vi "Lab Panel V5.23.vi"() -> ()   [LabVIEW 2013] (continued)
                    n2880 = Number To Decimal String(number=w5323) -> (decimal integer string=w5325:string)  [unwired: 1 in]
                    n2881 = Number To Decimal String(number=w5320) -> (decimal integer string=w5318:string)  [unwired: 1 in]
                    n2882 = Number To Decimal String(number=w5315) -> (decimal integer string=w5313:string)  [unwired: 1 in]
                    n2883 = Number To Decimal String(number=w5330) -> (decimal integer string=w5328:string)  [unwired: 1 in]
                    n2884 = Number To Decimal String(number=w5310) -> (decimal integer string=w5308:string)  [unwired: 1 in]
                    n2885 = Number To Decimal String(number=w5335) -> (decimal integer string=w5333:string)  [unwired: 1 in]
                    n2886 = Number To Decimal String(number=w5337) -> (decimal integer string=w5290:string)  [unwired: 1 in]
                    n2887 = Number To Decimal String(number=w5305) -> (decimal integer string=w5303:string)  [unwired: 1 in]
                    n2888 = Number To Decimal String(number=w5300) -> (decimal integer string=w5298:string)  [unwired: 1 in]
                    n2889 = Number To Decimal String(number=w5295) -> (decimal integer string=w5293:string)  [unwired: 1 in]
                    n2890 = Number To Fractional String(number=w5322, precision (6)=w5267) -> (F-format string=w5324:string)  [unwired: 2 in]
                    n2891 = Number To Fractional String(number=w5309, precision (6)=w5267) -> (F-format string=w5307:string)  [unwired: 2 in]
                    n2892 = Number To Fractional String(number=w5319, precision (6)=w5267) -> (F-format string=w5317:string)  [unwired: 2 in]
                    n2893 = Number To Fractional String(number=w5314, precision (6)=w5267) -> (F-format string=w5312:string)  [unwired: 2 in]
                    n2894 = Number To Fractional String(number=w5299, precision (6)=w5267) -> (F-format string=w5297:string)  [unwired: 2 in]
                    n2895 = Number To Fractional String(number=w5304, precision (6)=w5267) -> (F-format string=w5302:string)  [unwired: 2 in]
                    n2896 = Number To Fractional String(number=w5329, precision (6)=w5267) -> (F-format string=w5327:string)  [unwired: 2 in]
                    n2897 = Number To Fractional String(number=w5294, precision (6)=w5267) -> (F-format string=w5292:string)  [unwired: 2 in]
                    n2898 = Number To Fractional String(number=w5334, precision (6)=w5267) -> (F-format string=w5332:string)  [unwired: 2 in]
                    n2899 = Number To Fractional String(number=w5336, precision (6)=w5267) -> (F-format string=w5289:string)  [unwired: 2 in]
                    n2900 = Concatenate Strings(w5266, w5308, w5266, w5307, w5266, w5306) -> (w5282:string)
                    n2901 = Concatenate Strings(w5266, w5303, w5266, w5302, w5266, w5301) -> (w5281:string)
                    n2902 = Concatenate Strings(w5266, w5298, w5266, w5297, w5266, w5296) -> (w5280:string)
                    n2903 = Concatenate Strings(w5266, w5293, w5266, w5292, w5266, w5291) -> (w5279:string)
                    n2904 = Concatenate Strings(w5266, w5290, w5266, w5289, w5266, w5288) -> (w5278:string)
                    n2905 = Concatenate Strings(w5266, w5333, w5266, w5332, w5266, w5331) -> (w5287:string)
                    n2906 = Concatenate Strings(w5266, w5313, w5266, w5312, w5266, w5311) -> (w5283:string)
                    n2907 = Concatenate Strings(w5266, w5328, w5266, w5327, w5266, w5326) -> (w5286:string)
                    n2908 = Concatenate Strings(w5266, w5325, w5266, w5324, w5266, w5321) -> (w5285:string)
                    n2909 = Concatenate Strings(w5266, w5318, w5266, w5317, w5266, w5316) -> (w5284:string)
                    n2910 = Concatenate Strings("]", "\r") -> (w5263:string)
                    n2911 = Concatenate Strings(w5258, w5283, w5263) -> (w5273:string)
                    n2912 = Concatenate Strings(w5260, w5285, w5263) -> (w5275:string)
                    n2913 = Concatenate Strings(w5259, w5284, w5263) -> (w5274:string)
                    n2914 = Concatenate Strings(w5255, w5280, w5263) -> (w5270:string)
                    n2915 = Concatenate Strings(w5256, w5279, w5263) -> (w5271:string)
                    n2916 = Concatenate Strings(w5254, w5281, w5263) -> (w5269:string)
                    n2917 = Concatenate Strings(w5253, w5282, w5263) -> (w5268:string)
                    n2918 = Concatenate Strings(w5257, w5278, w5263) -> (w5272:string)
                    n2919 = Concatenate Strings(w5261, w5286, w5263) -> (w5276:string)
                    n2920 = Concatenate Strings(w5262, w5287, w5263) -> (w5277:string)
                    n2921 = Concatenate Strings(w5277, w5276, w5275, w5274, w5273, w5268, w5269, w5270, w5271, w5272) -> (w5246:string)
                    n2922 = Concatenate Strings("[PANEL/", "DESC/", "CYCLES/", "MINS/", "STATUS]", "\r", w5246) -> (w5245:string)
                    "MAIL REPORT" <- w5245
                    n2923 = global write "Global display 3.vi" "log all"(w5245) -> ()
                  }
                  frame #2 {
                    w5376 = "END"
                    n2924 = local read "mail control"() -> (w5377:string)
                    n2925 = case shown="False" w5372 {
                      tunnel: w5377 -> [w5401 _]
                      tunnel: w5376 -> [w5400 _]
                      tunnel: [w5399 FALSE] -> w5362
                      frame False {
                        n2926 = Equal?(x=w5401, y=w5400) -> (x = y?=w5399:bool)
                      }
                      frame True {
                      }
                    }
                    n2927 = case shown="False" w5378 {
                      tunnel: w5377 -> [w5417 _]
                      tunnel: w5376 -> [w5416 _]
                      tunnel: [w5415 FALSE] -> w5366
                      frame False {
                        n2928 = Equal?(x=w5417, y=w5416) -> (x = y?=w5415:bool)
                      }
                      frame True {
                      }
                    }
                    n2929 = case shown="False" w5375 {
                      tunnel: w5377 -> [w5413 _]
                      tunnel: w5376 -> [w5412 _]
                      tunnel: [w5411 FALSE] -> w5365
                      frame False {
                        n2930 = Equal?(x=w5413, y=w5412) -> (x = y?=w5411:bool)
                      }
                      frame True {
                      }
                    }
                    n2931 = case shown="False" w5373 {
                      tunnel: w5377 -> [w5405 _]
                      tunnel: w5376 -> [w5404 _]
                      tunnel: [w5403 FALSE] -> w5363
                      frame False {
                        n2932 = Equal?(x=w5405, y=w5404) -> (x = y?=w5403:bool)
                      }
                      frame True {
                      }
                    }
                    n2933 = case shown="False" w5374 {
                      tunnel: w5377 -> [w5409 _]
                      tunnel: w5376 -> [w5408 _]
                      tunnel: [w5407 FALSE] -> w5364
                      frame False {
                        n2934 = Equal?(x=w5409, y=w5408) -> (x = y?=w5407:bool)
                      }
                      frame True {
                      }
                    }
                    n2935 = Or(x=w5364, y=w5363) -> (x .or. y?=w5355:bool)
                    n2936 = Or(x=w5366, y=w5365) -> (x .or. y?=w5356:bool)
                    n2937 = Or(x=w5356, y=w5355) -> (x .or. y?=w5351:bool)
                    n2938 = case shown="False" w5368 {
                      tunnel: w5377 -> [w5385 _]
                      tunnel: w5376 -> [w5384 _]
                      tunnel: [w5383 FALSE] -> w5357
                      frame False {
                        n2939 = Equal?(x=w5385, y=w5384) -> (x = y?=w5383:bool)
                      }
                      frame True {
                      }
                    }
                    n2940 = case shown="False" w5367 {
                      tunnel: w5377 -> [w5381 _]
                      tunnel: w5376 -> [w5380 _]
                      tunnel: [w5379 FALSE] -> w5361
                      frame False {
                        n2941 = Equal?(x=w5381, y=w5380) -> (x = y?=w5379:bool)
                      }
                      frame True {
                      }
                    }
                    n2942 = case shown="False" w5369 {
                      tunnel: w5377 -> [w5389 _]
                      tunnel: w5376 -> [w5388 _]
                      tunnel: [w5387 FALSE] -> w5358
                      frame False {
                        n2943 = Equal?(x=w5389, y=w5388) -> (x = y?=w5387:bool)
                      }
                      frame True {
                      }
                    }
                    n2944 = case shown="False" w5371 {
                      tunnel: w5377 -> [w5397 _]
                      tunnel: w5376 -> [w5396 _]
                      tunnel: [w5395 FALSE] -> w5360
                      frame False {
                        n2945 = Equal?(x=w5397, y=w5396) -> (x = y?=w5395:bool)
                      }
                      frame True {
                      }
                    }
                    n2946 = case shown="False" w5370 {
                      tunnel: w5377 -> [w5393 _]
                      tunnel: w5376 -> [w5392 _]
                      tunnel: [w5391 FALSE] -> w5359
                      frame False {
                        n2947 = Equal?(x=w5393, y=w5392) -> (x = y?=w5391:bool)
                      }
                      frame True {
                      }
                    }
                    n2948 = Or(x=w5360, y=w5359) -> (x .or. y?=w5354:bool)
                    n2949 = Or(x=w5358, y=w5357) -> (x .or. y?=w5353:bool)
                    n2950 = Or(x=w5361, y=w5362) -> (x .or. y?=w5349:bool)
                    n2951 = Or(x=w5354, y=w5353) -> (x .or. y?=w5352:bool)
                    n2952 = Or(x=w5351, y=w5352) -> (x .or. y?=w5350:bool)
                    n2953 = Or(x=w5350, y=w5349) -> (x .or. y?=w5348:bool)
                  }
                  frame #3 {
                    n2954 = local read "on loops"() -> (w5431:dbl)
                    n2955 = local read "jig cycle"() -> (w5428:dbl)
                    n2956 = local read "Send Mail Now"() -> (w5422:bool)
                    n2957 = Add(x=w5431, y=3.0) -> (x+y=w5429:dbl)
                    n2958 = Equal?(x=w5428, y=w5429) -> (x = y?=w5423:bool)
                    n2959 = And(x=w5423, y=w5422) -> (x .and. y?=w5421:bool)
                    n2960 = And(x=w5427, y=w5423) -> (x .and. y?=w5426:bool)
                    n2961 = And(x=w5426, y=w5425) -> (x .and. y?=w5424:bool)
                    n2962 = Or(x=w5424, y=w5421) -> (x .or. y?=w5420:bool)
                    n2963 = case shown="True" w5420 {
                      tunnel: w5436 -> [_ w5442]
                      tunnel: w5435 -> [_ w5441]
                      tunnel: "Lab Panel Test Status" -> [_ w5440]
                      tunnel: w5433 -> [_ w5439]
                      tunnel: w5432 -> [_ w5438]
                      tunnel: w5419 -> [_ w5437]
                      frame False {
                      }
                      frame True {
                        n2964 = stacked-sequence {
                          tunnel: w5442 -> [w5450 _]
                          tunnel: w5441 -> [w5449 _]
                          tunnel: w5440 -> [w5448 _]
                          tunnel: w5439 -> [w5447 _]
                          tunnel: w5438 -> [w5446 _]
                          tunnel: w5437 -> [w5445 _]
                          frame #0 {
                            n2965 = call "sub vi - send mail v5.vi"("TO:"=w5450, "subject"=w5448, "from"=w5446, "out going server"=w5447, "message"=w5449) -> ("error out"=w5444:errorcluster)  [unwired: 10 in]
                            n2966 = Bundle(cluster=w5445, "mail error"=w5444) -> (w5443:T7)  [unwired: 6 in]
                            n2967 = local write "MAIL SETTINGS"(w5443) -> ()
                          }
                          frame #1 {
                            n2968 = local write "mail control"("") -> ()
                            n2969 = local write "Send Mail Now"(FALSE) -> ()
                          }
                        }
                      }
                    }
                  }
                }
              }
            }
          }
          frame #18 {
            # "save jig cycle values once all run switches are off"
            n2970 = stacked-sequence {
              tunnel: w5462 -> [_ w5491]
              tunnel: w5461 -> [_ w5490]
              tunnel: w5460 -> [_ w5489]
              tunnel: w5459 -> [_ w5488]
              tunnel: w5458 -> [_ w5487]
              tunnel: w5457 -> [_ w5486]
              tunnel: w5456 -> [_ w5485]
              tunnel: w5455 -> [_ w5484]
              tunnel: w5454 -> [_ w5483]
              tunnel: w5453 -> [_ w5482]
              frame #0 {
              }
              frame #1 {
                n2971 = Not(x=w5482) -> (.not. x?=w5465:bool)
                n2972 = Not(x=w5490) -> (.not. x?=w5480:bool)
                n2973 = Not(x=w5487) -> (.not. x?=w5475:bool)
                n2974 = Not(x=w5485) -> (.not. x?=w5471:bool)
                n2975 = Not(x=w5483) -> (.not. x?=w5467:bool)
                n2976 = Not(x=w5491) -> (.not. x?=w5481:bool)
                n2977 = Not(x=w5489) -> (.not. x?=w5479:bool)
                n2978 = Not(x=w5486) -> (.not. x?=w5473:bool)
                n2979 = Not(x=w5488) -> (.not. x?=w5477:bool)
                n2980 = Not(x=w5484) -> (.not. x?=w5469:bool)
                n2981 = local read "Save JC"() -> (w5493:bool)
                n2982 = And(x=w5481, y=w5480) -> (x .and. y?=w5478:bool)
                n2983 = And(x=w5478, y=w5479) -> (x .and. y?=w5476:bool)
                n2984 = And(x=w5476, y=w5477) -> (x .and. y?=w5474:bool)
                n2985 = And(x=w5474, y=w5475) -> (x .and. y?=w5472:bool)
                n2986 = And(x=w5472, y=w5473) -> (x .and. y?=w5470:bool)
                n2987 = And(x=w5470, y=w5471) -> (x .and. y?=w5468:bool)
                n2988 = And(x=w5468, y=w5469) -> (x .and. y?=w5466:bool)
                n2989 = And(x=w5466, y=w5467) -> (x .and. y?=w5464:bool)
                n2990 = And(x=w5464, y=w5465) -> (x .and. y?=w5463:bool)
                n2991 = And(x=w5463, y=w5493) -> (x .and. y?=w5492:bool)
                n2992 = case shown="True" w5492 {
                  tunnel: w5463 -> [w5494 _]
                  frame False {
                    n2993 = case shown="False" w5494 {
                      frame False {
                        n2994 = local write "Save JC"(TRUE) -> ()
                      }
                      frame True {
                      }
                    }
                  }
                  frame True {
                    n2995 = stacked-sequence {
                      frame #0 {
                        n2996 = String To Path(string="c:\\crabtree\\Jig Cycles\\") -> (path=w5506:path)
                        n2997 = Build Path(base path=w5506, name or relative path="jigcycles.bin") -> (appended path=w5504:path)
                        n2998 = Create Folder(path (use dialog)=w5506) -> (error out=w5508:errorcluster)  [unwired: 2 in, 2 out]
                        n2999 = local read "JIG RELAY CYCLES"() -> (w5498:T8)
                        n3000 = call <vilib>:"Clear Errors.vi"("error in (no error)"=w5508) -> ()  [unwired: 6 in, 1 out]
                        n3001 = local write "Save JC"(FALSE) -> ()
                        n3002 = Open/Create/Replace File(file path (use dialog)=w5504, operation (0:open)=T17."replace or create") -> (refnum out=w5502:refnum<file>, error out=w5503:errorcluster)  [unwired: 4 in, 1 out]
                        n3003 = Write to Binary File(file (use dialog)=w5502, data=w5498, error in=w5503) -> (refnum out=w5501:refnum<file>, error out=w5500:errorcluster)  [unwired: 3 in, 1 out]
                        n3004 = Close File(refnum=w5501, error in=w5500) -> (error out=w5499:errorcluster)  [unwired: 1 out]
                        n3005 = local write "data file error"(w5499) -> ()
                      }
                      frame #1 {
                        n3006 = local read "JIG RELAY CYCLES"() -> (w5531:T8)
                        n3007 = Unbundle By Name(w5531) -> ("LAB01-1"=w5526:dbl, "LAB01-2"=w5525:dbl, "LAB02-1"=w5523:dbl, "LAB02-2"=w5522:dbl, "LAB03-1"=w5520:dbl, "LAB03-2"=w5517:dbl, "LAB04-1"=w5516:dbl, "LAB04-2"=w5514:dbl, "LAB05-1"=w5512:dbl, "LAB05-2"=w5510:dbl)
                        n3008 = stacked-sequence {
                          tunnel: w5526 -> [w5534 _ _ _ _ _ _ _ _ _]
                          tunnel: 1000000 -> [w5537 w5547 w5557 w5567 w5577 w5587 w5597 w5607 w5617 w5627]
                          tunnel: [w5535 _ _ _ _ _ _ _ _ _] -> w5529
                          tunnel: "TEST STATION HAS REACHED 1 MILLION CYCLES, REPLACE  CONTROL RELAYS" -> [w5533 w5545 w5555 w5565 w5575 w5585 w5595 w5605 w5615 w5625]
                          tunnel: [_ w5544 _ _ _ _ _ _ _ _] -> w5527
                          tunnel: w5525 -> [_ w5543 _ _ _ _ _ _ _ _]
                          tunnel: [_ _ w5554 _ _ _ _ _ _ _] -> w5524
                          tunnel: w5523 -> [_ _ w5553 _ _ _ _ _ _ _]
                          tunnel: w5522 -> [_ _ _ w5564 _ _ _ _ _ _]
                          tunnel: [_ _ _ w5563 _ _ _ _ _ _] -> w5521
                          tunnel: w5520 -> [_ _ _ _ w5574 _ _ _ _ _]
                          tunnel: [_ _ _ _ w5573 _ _ _ _ _] -> w5519
                          tunnel: [_ _ _ _ _ w5584 _ _ _ _] -> w5518
                          tunnel: w5517 -> [_ _ _ _ _ w5583 _ _ _ _]
                          tunnel: w5516 -> [_ _ _ _ _ _ w5594 _ _ _]
                          tunnel: [_ _ _ _ _ _ w5593 _ _ _] -> w5515
                          tunnel: w5514 -> [_ _ _ _ _ _ _ w5604 _ _]
                          tunnel: [_ _ _ _ _ _ _ w5603 _ _] -> w5513
                          tunnel: w5512 -> [_ _ _ _ _ _ _ _ w5614 _]
                          tunnel: [_ _ _ _ _ _ _ _ w5613 _] -> w5511
                          tunnel: w5510 -> [_ _ _ _ _ _ _ _ _ w5624]
                          tunnel: [_ _ _ _ _ _ _ _ _ w5623] -> w5509
                          frame #0 {
                            n3009 = Greater?(x=w5534, y=w5537) -> (0:w5536:bool)
                            n3010 = case shown="True" w5536 {
                              tunnel: [w5538 0] -> w5535
                              tunnel: w5534 -> [w5538 _]
                              tunnel: w5533 -> [_ w5539]
                              frame False {
                              }
                              frame True {
                                n3011 = Concatenate Strings("LA01-1 ", w5539) -> (w5542:string)
                                n3012 = One Button Dialog(message=w5542) -> ()  [unwired: 1 in, 1 out]
                              }
                            }
                          }
                          frame #1 {
                            n3013 = Greater?(x=w5543, y=w5547) -> (0:w5546:bool)
                            n3014 = case shown="True" w5546 {
                              tunnel: [w5548 0] -> w5544
                              tunnel: w5543 -> [w5548 _]
                              tunnel: w5545 -> [_ w5549]
                              frame False {
                              }
                              frame True {
                                n3015 = Concatenate Strings("LA01-2 ", w5549) -> (w5552:string)
                                n3016 = One Button Dialog(message=w5552) -> ()  [unwired: 1 in, 1 out]
                              }
                            }
                          }
                          frame #2 {
                            n3017 = Greater?(x=w5553, y=w5557) -> (0:w5556:bool)
                            n3018 = case shown="True" w5556 {
                              tunnel: [w5558 0] -> w5554
                              tunnel: w5553 -> [w5558 _]
                              tunnel: w5555 -> [_ w5559]
                              frame False {
                              }
                              frame True {
                                n3019 = Concatenate Strings("LA02-1 ", w5559) -> (w5562:string)
                                n3020 = One Button Dialog(message=w5562) -> ()  [unwired: 1 in, 1 out]
                              }
                            }
                          }
                          frame #3 {
                            n3021 = Greater?(x=w5564, y=w5567) -> (0:w5566:bool)
                            n3022 = case shown="True" w5566 {
                              tunnel: [w5568 0] -> w5563
                              tunnel: w5564 -> [w5568 _]
                              tunnel: w5565 -> [_ w5569]
                              frame False {
                              }
                              frame True {
                                n3023 = Concatenate Strings("LA02-2 ", w5569) -> (w5572:string)
                                n3024 = One Button Dialog(message=w5572) -> ()  [unwired: 1 in, 1 out]
                              }
                            }
                          }
                          frame #4 {
                            n3025 = Greater?(x=w5574, y=w5577) -> (0:w5576:bool)
                            n3026 = case shown="True" w5576 {
                              tunnel: [w5578 0] -> w5573
                              tunnel: w5574 -> [w5578 _]
                              tunnel: w5575 -> [_ w5579]
                              frame False {
                              }
                              frame True {
                                n3027 = Concatenate Strings("LA03-1 ", w5579) -> (w5582:string)
                                n3028 = One Button Dialog(message=w5582) -> ()  [unwired: 1 in, 1 out]
                              }
                            }
                          }
                          frame #5 {
                            n3029 = Greater?(x=w5583, y=w5587) -> (0:w5586:bool)
                            n3030 = case shown="True" w5586 {
                              tunnel: [w5588 0] -> w5584
                              tunnel: w5583 -> [w5588 _]
                              tunnel: w5585 -> [_ w5589]
                              frame False {
                              }
                              frame True {
                                n3031 = Concatenate Strings("LA03-2 ", w5589) -> (w5592:string)
                                n3032 = One Button Dialog(message=w5592) -> ()  [unwired: 1 in, 1 out]
                              }
                            }
                          }
                          frame #6 {
                            n3033 = Greater?(x=w5594, y=w5597) -> (0:w5596:bool)
                            n3034 = case shown="True" w5596 {
                              tunnel: [w5598 0] -> w5593
                              tunnel: w5594 -> [w5598 _]
                              tunnel: w5595 -> [_ w5599]
                              frame False {
                              }
                              frame True {
                                n3035 = Concatenate Strings("LA04-1 ", w5599) -> (w5602:string)
                                n3036 = One Button Dialog(message=w5602) -> ()  [unwired: 1 in, 1 out]
                              }
                            }
                          }
                          frame #7 {
                            n3037 = Greater?(x=w5604, y=w5607) -> (0:w5606:bool)
                            n3038 = case shown="True" w5606 {
                              tunnel: [w5608 0] -> w5603
                              tunnel: w5604 -> [w5608 _]
                              tunnel: w5605 -> [_ w5609]
                              frame False {
                              }
                              frame True {
                                n3039 = Concatenate Strings("LA04-2 ", w5609) -> (w5612:string)
                                n3040 = One Button Dialog(message=w5612) -> ()  [unwired: 1 in, 1 out]
                              }
                            }
                          }
                          frame #8 {
                            n3041 = Greater?(x=w5614, y=w5617) -> (0:w5616:bool)
                            n3042 = case shown="True" w5616 {
                              tunnel: [w5618 0] -> w5613
                              tunnel: w5614 -> [w5618 _]
                              tunnel: w5615 -> [_ w5619]
                              frame False {
                              }
                              frame True {
                                n3043 = Concatenate Strings("LA05-1 ", w5619) -> (w5622:string)
                                n3044 = One Button Dialog(message=w5622) -> ()  [unwired: 1 in, 1 out]
                              }
                            }
                          }
                          frame #9 {
                            n3045 = Greater?(x=w5624, y=w5627) -> (0:w5626:bool)
                            n3046 = case shown="True" w5626 {
                              tunnel: [w5628 0] -> w5623
                              tunnel: w5624 -> [w5628 _]
                              tunnel: w5625 -> [_ w5629]
                              frame False {
                              }
                              frame True {
                                n3047 = Concatenate Strings("LA05-2 ", w5629) -> (w5632:string)
                                n3048 = One Button Dialog(message=w5632) -> ()  [unwired: 1 in, 1 out]
                              }
                            }
                          }
                        }
                        n3049 = Bundle By Name(cluster=w5531, "LAB01-1"=w5529, "LAB01-2"=w5527, "LAB02-1"=w5524, "LAB02-2"=w5521, "LAB03-1"=w5519, "LAB03-2"=w5518, "LAB04-1"=w5515, "LAB04-2"=w5513, "LAB05-1"=w5511, "LAB05-2"=w5509) -> (w5530:T8)
                        n3050 = local write "JIG RELAY CYCLES"(w5530) -> ()
                      }
                    }
                  }
                }
              }
            }
          }
          frame #19 {
            # "get temperature values"
            n3051 = local read "Panel #"() -> (w5633:dbl)
            n3052 = local read "Simulate"() -> (w5646:bool)
            n3053 = local read "Temp Test Cal"() -> (w5643:dbl)
            n3054 = stacked-sequence {
              seq-local: [w5649 _] -> [_ w5742]
              tunnel: w5646 -> [_ w5756]
              tunnel: T14 {"1  (A) cal"=1.0, "1 (V) cal"=1.0, "1 (PF) cal"=1.0, "1 (TL) cal"=1.0, "1 (TN) cal"=1.0, "2 (A) cal"=1.0, "2 (V) cal"=1.0, "2 (PF) cal"=1.0, "2 (TL) cal"=1.0, "2 (TN) cal"=1.0} ("CAL LAB01") -> [_ w5755]
              tunnel: w5644 -> [_ w5754]
              tunnel: w5643 -> [_ w5753]
              tunnel: w5642 -> [_ w5752]
              tunnel: w5641 -> [_ w5751]
              tunnel: w5640 -> [_ w5750]
              tunnel: w5639 -> [_ w5749]
              tunnel: w5638 -> [_ w5748]
              tunnel: w5637 -> [_ w5747]
              tunnel: w5636 -> [_ w5746]
              tunnel: w5635 -> [_ w5745]
              tunnel: w5634 -> [_ w5744]
              tunnel: w5633 -> [_ w5743]
              frame #0 {
                # "only get temperature from initial valid temperature circuits"
                n3055 = local read "Select COM port"() -> (w5650:refnum<visa-resource-name>)
                "COM port" <- w5650
                n3056 = global write "Global 1.vi" "COM port"(w5650) -> ()
                n3057 = global write "Global 1.vi" "tmp dly lps"("Temp Delay Lps") -> ()
                n3058 = global write "Global 1.vi" "dly value"("Temp Value") -> ()
                n3059 = local read "jig cycle"() -> (w5652:dbl)
                n3060 = local read "on loops"() -> (w5654:dbl)
                n3061 = Add(x=w5654, y=3) -> (x+y=w5655:dbl)
                n3062 = local read "Panel #"() -> (w5651:dbl)
                n3063 = Equal?(x=w5652, y=w5655) -> (x = y?=w5649:bool)
                n3064 = stacked-sequence {
                  tunnel: w5651 -> [w5657 _]
                  tunnel: w5649 -> [w5656 _]
                  frame #0 {
                    n3065 = case shown="True" w5656 {
                      tunnel: w5657 -> [_ w5661]
                      frame False {
                      }
                      frame True {
                        n3066 = local read "Simulate"() -> (w5658:bool)
                        n3067 = case shown="1" w5661 {
                          tunnel: 1.0 -> [_ w5664 w5677 w5690 w5702 w5716]
                          tunnel: w5658 -> [_ w5663 w5676 w5689 w5703 w5715]
                          frame 0, Default {
                            (unwired) FALSE
                          }
                          frame 1 {
                            n3068 = local read "LAB01-TP"() -> (w5662:bool)
                            n3069 = case shown="True" w5662 {
                              tunnel: w5664 -> [_ w5674]
                              tunnel: w5663 -> [_ w5670]
                              frame False {
                              }
                              frame True {
                                w5672 = FALSE
                                n3070 = local read "Temp Er 01"() -> (w5667:dbl)
                                n3071 = call "sub vi - GET ALL TEMP v7.vi"("LA01-EN"=TRUE, "simulate"=w5670, "LA02-EN"=w5672, "LA03-EN"=w5672, "LA04-EN"=w5672, "LA05-EN"=w5672, "Gen Cal Value"=w5674) -> ("LA01 TEMP"=w5671:T25, "error"=w5669:bool)  [unwired: 2 in, 5 out]
                                n3072 = Increment(x=w5667) -> (x+1=w5666:dbl)
                                n3073 = local write "LAB01 TEMP"(w5671) -> ()
                                n3074 = Select(t=w5666, s=w5669, f=0.0) -> (s? t:f=→"Temp Er 01":dbl)
                              }
                            }
                          }
                          frame 2 {
                            n3075 = local read "LAB02-TP"() -> (w5675:bool)
                            n3076 = case shown="True" w5675 {
                              tunnel: w5677 -> [_ w5684]
                              tunnel: w5676 -> [_ w5683]
                              frame False {
                              }
                              frame True {
                                w5685 = FALSE
                                n3077 = local read "Temp Er 02"() -> (w5680:dbl)
                                n3078 = call "sub vi - GET ALL TEMP v7.vi"("LA01-EN"=w5685, "simulate"=w5683, "LA02-EN"=TRUE, "LA03-EN"=w5685, "LA04-EN"=w5685, "LA05-EN"=w5685, "Gen Cal Value"=w5684) -> ("LA02 TEMP"=w5687:T25, "error"=w5681:bool)  [unwired: 2 in, 5 out]
                                n3079 = Increment(x=w5680) -> (x+1=w5679:dbl)
                                n3080 = local write "LAB02 TEMP"(w5687) -> ()
                                n3081 = Select(t=w5679, s=w5681, f=0.0) -> (s? t:f=→"Temp Er 02":dbl)
                              }
                            }
                          }
                          frame 3 {
                            n3082 = local read "LAB03-TP"() -> (w5688:bool)
                            n3083 = case shown="True" w5688 {
                              tunnel: w5690 -> [_ w5698]
                              tunnel: w5689 -> [_ w5696]
                              frame False {
                              }
                              frame True {
                                w5699 = FALSE
                                n3084 = local read "Temp Er 03"() -> (w5694:dbl)
                                n3085 = call "sub vi - GET ALL TEMP v7.vi"("LA01-EN"=w5699, "simulate"=w5696, "LA02-EN"=w5699, "LA03-EN"=TRUE, "LA04-EN"=w5699, "LA05-EN"=w5699, "Gen Cal Value"=w5698) -> ("LA03 TEMP"=w5697:T25, "error"=w5692:bool)  [unwired: 2 in, 5 out]
                                n3086 = Increment(x=w5694) -> (x+1=w5693:dbl)
                                n3087 = local write "LAB03 TEMP"(w5697) -> ()
                                n3088 = Select(t=w5693, s=w5692, f=0.0) -> (s? t:f=→"Temp Er 03":dbl)
                              }
                            }
                          }
                          frame 4 {
                            n3089 = local read "LAB04-TP"() -> (w5701:bool)
                            n3090 = case shown="True" w5701 {
                              tunnel: w5703 -> [_ w5711]
                              tunnel: w5702 -> [_ w5710]
                              frame False {
                              }
                              frame True {
                                w5712 = FALSE
                                n3091 = local read "Temp Er 04"() -> (w5708:dbl)
                                n3092 = call "sub vi - GET ALL TEMP v7.vi"("LA01-EN"=w5712, "simulate"=w5711, "LA02-EN"=w5712, "LA03-EN"=w5712, "LA04-EN"=TRUE, "LA05-EN"=w5712, "Gen Cal Value"=w5710) -> ("LA04 TEMP"=w5709:T25, "error"=w5705:bool)  [unwired: 2 in, 5 out]
                                n3093 = Increment(x=w5708) -> (x+1=w5706:dbl)
                                n3094 = local write "LAB04 TEMP"(w5709) -> ()
                                n3095 = Select(t=w5706, s=w5705, f=0.0) -> (s? t:f=→"Temp Er 04":dbl)
                              }
                            }
                          }
                          frame 5 {
                            n3096 = local read "LAB05-TP"() -> (w5714:bool)
                            n3097 = case shown="True" w5714 {
                              tunnel: w5716 -> [_ w5723]
                              tunnel: w5715 -> [_ w5722]
                              frame False {
                              }
                              frame True {
                                w5725 = FALSE
                                n3098 = local read "Temp Er 05"() -> (w5719:dbl)
                                n3099 = call "sub vi - GET ALL TEMP v7.vi"("LA01-EN"=w5725, "simulate"=w5722, "LA02-EN"=w5725, "LA03-EN"=w5725, "LA04-EN"=w5725, "LA05-EN"=TRUE, "Gen Cal Value"=w5723) -> ("error"=w5721:bool, "LA05 TEMP"=w5724:T25)  [unwired: 2 in, 5 out]
                                n3100 = local write "LAB05 TEMP"(w5724) -> ()
                                n3101 = Increment(x=w5719) -> (x+1=w5720:dbl)
                                n3102 = Select(t=w5720, s=w5721, f=0.0) -> (s? t:f=→"Temp Er 05":dbl)
                              }
                            }
                          }
                        }
                        n3103 = local write "TEMP"(TRUE) -> ()
                      }
                    }
                  }
                  frame #1 {
                    w5727 = 5
                    n3104 = local read "Temp Er 05"() -> (w5737:dbl)
                    n3105 = local read "Temp Er 03"() -> (w5739:dbl)
                    n3106 = local read "Temp Er 04"() -> (w5738:dbl)
                    n3107 = local read "Temp Er 01"() -> (w5741:dbl)
                    n3108 = local read "Temp Er 02"() -> (w5740:dbl)
                    n3109 = Greater Or Equal?(x=w5738, y=w5727) -> (x >= y?=w5731:bool)
                    n3110 = Greater Or Equal?(x=w5740, y=w5727) -> (x >= y?=w5733:bool)
                    n3111 = Greater Or Equal?(x=w5739, y=w5727) -> (x >= y?=w5732:bool)
                    n3112 = Greater Or Equal?(x=w5737, y=w5727) -> (x >= y?=w5730:bool)
                    n3113 = Greater Or Equal?(x=w5741, y=w5727) -> (x >= y?=w5734:bool)
                    n3114 = Or(x=w5732, y=w5731) -> (x .or. y?=w5735:bool)
                    n3115 = Or(x=w5734, y=w5733) -> (x .or. y?=w5736:bool)
                    n3116 = Or(x=w5736, y=w5735) -> (x .or. y?=w5729:bool)
                    n3117 = Or(x=w5729, y=w5730) -> (x .or. y?=→"Error Temp":bool)
                  }
                }
              }
              frame #1 {
                n3118 = case shown="True" w5742 {
                  tunnel: w5756 -> [_ w5770]
                  tunnel: w5755 -> [_ w5769]
                  tunnel: w5754 -> [_ w5768]
                  tunnel: w5753 -> [_ w5767]
                  tunnel: w5752 -> [_ w5766]
                  tunnel: w5751 -> [_ w5765]
                  tunnel: w5750 -> [_ w5764]
                  tunnel: w5749 -> [_ w5763]
                  tunnel: w5748 -> [_ w5762]
                  tunnel: w5747 -> [_ w5761]
                  tunnel: w5746 -> [_ w5760]
                  tunnel: w5745 -> [_ w5759]
                  tunnel: w5744 -> [_ w5758]
                  tunnel: w5743 -> [_ w5757]
                  frame False {
                  }
                  frame True {
                    n3119 = case shown="2" w5757 {
                      tunnel: w5770 -> [_ w5783 w5828 w5873 w5918 w5963]
                      tunnel: w5769 -> [_ w5782 w5827 w5872 w5917 w5962]
                      tunnel: w5768 -> [_ w5772 _ _ _ _]
                      tunnel: w5767 -> [_ w5777 w5826 w5871 w5916 w5961]
                      tunnel: w5766 -> [_ w5771 _ _ _ _]
                      tunnel: w5765 -> [_ _ w5817 _ _ _]
                      tunnel: w5764 -> [_ _ w5816 _ _ _]
                      tunnel: w5763 -> [_ _ _ w5862 _ _]
                      tunnel: w5762 -> [_ _ _ w5861 _ _]
                      tunnel: w5761 -> [_ _ _ _ w5907 _]
                      tunnel: w5760 -> [_ _ _ _ w5906 _]
                      tunnel: w5759 -> [_ _ _ _ _ w5952]
                      tunnel: w5758 -> [_ _ _ _ _ w5951]
                      frame ..0 {
                      }
                      frame 1 {
                        n3120 = case shown="False" w5783 {
                          tunnel: [w5814 w5815] -> w5799
                          tunnel: w5782 -> [_ w5815]
                          frame False {
                            n3121 = local read "CAL LAB01"() -> (w5814:T14)
                          }
                          frame True {
                          }
                        }
                        n3122 = local read "TEMP LA01"() -> (w5790:T9)
                        n3123 = local read "LAB01 TEMP"() -> (w5789:T12)
                        n3124 = call "sub vi - temperature delay v3.vi"("2-run"=w5771, "1-run"=w5772, "temp values IN"=w5790, "temp signals"=w5789) -> ("T2-N"=w5785:dbl, "T2-L"=w5786:dbl, "T1-N"=w5787:dbl, "T1-L"=w5788:dbl, "temp values OUT"=w5784:T44)  [unwired: 3 in]
                        n3125 = Unbundle By Name(w5799) -> ("1 (TL) cal"=w5794:dbl, "1 (TN) cal"=w5793:dbl, "2 (TL) cal"=w5792:dbl, "2 (TN) cal"=w5791:dbl)  [unwired: 6 out]
                        n3126 = local write "TEMP LA01"(w5784) -> ()
                        n3127 = Multiply(x=w5788, y=w5794) -> (x*y=w5781:dbl)
                        n3128 = Multiply(x=w5787, y=w5793) -> (x*y=w5779:dbl)
                        n3129 = Multiply(x=w5786, y=w5792) -> (x*y=w5776:dbl)
                        n3130 = Multiply(x=w5785, y=w5791) -> (x*y=w5775:dbl)
                        n3131 = case shown="True" w5772 {
                          tunnel: w5781 -> [w5808 w5813]
                          tunnel: w5777 -> [_ w5811]
                          tunnel: [w5808 w5812] -> w5780
                          tunnel: w5779 -> [w5807 w5810]
                          tunnel: [w5807 w5809] -> w5778
                          frame False {
                          }
                          frame True {
                            n3132 = Multiply(x=w5811, y=w5810) -> (x*y=w5809:dbl)
                            n3133 = Multiply(x=w5811, y=w5813) -> (x*y=w5812:dbl)
                          }
                        }
                        n3134 = case shown="True" w5771 {
                          tunnel: w5776 -> [w5801 w5806]
                          tunnel: w5777 -> [_ w5804]
                          tunnel: [w5801 w5805] -> w5774
                          tunnel: w5775 -> [w5800 w5803]
                          tunnel: [w5800 w5802] -> w5773
                          frame False {
                          }
                          frame True {
                            n3135 = Multiply(x=w5804, y=w5803) -> (x*y=w5802:dbl)
                            n3136 = Multiply(x=w5804, y=w5806) -> (x*y=w5805:dbl)
                          }
                        }
                        n3137 = local read "SIG LAB01-2"() -> (w5796:T2)
                        n3138 = local read "SIG LAB01-1"() -> (w5798:T2)
                        n3139 = Bundle By Name(cluster=w5798, "Tmp Live"=w5780, "Tmp Neut"=w5778) -> (w5797:T2)
                        n3140 = Bundle By Name(cluster=w5796, "Tmp Live"=w5774, "Tmp Neut"=w5773) -> (w5795:T2)
                        n3141 = local write "SIG LAB01-1"(w5797) -> ()
                        n3142 = local write "SIG LAB01-2"(w5795) -> ()
                      }
                      frame 2 {
                        n3143 = case shown="True" w5828 {
                          tunnel: [w5859 w5860] -> w5844
                          tunnel: w5827 -> [_ w5860]
                          frame False {
                            n3144 = local read "CAL LAB02"() -> (w5859:T15)
                          }
                          frame True {
                          }
                        }
                        n3145 = local read "LAB02 TEMP"() -> (w5835:T12)
                        n3146 = local read "TEMP LA02"() -> (w5834:T9)
                        n3147 = call "sub vi - temperature delay v3.vi"("2-run"=w5816, "1-run"=w5817, "temp values IN"=w5834, "temp signals"=w5835) -> ("T2-N"=w5829:dbl, "T2-L"=w5830:dbl, "T1-N"=w5831:dbl, "T1-L"=w5832:dbl, "temp values OUT"=w5833:T44)  [unwired: 3 in]
                        n3148 = Unbundle By Name(w5844) -> ("1 (TL) cal"=w5839:dbl, "1 (TN) cal"=w5838:dbl, "2 (TL) cal"=w5837:dbl, "2 (TN) cal"=w5836:dbl)  [unwired: 6 out]
                        n3149 = local write "TEMP LA02"(w5833) -> ()
                        n3150 = Multiply(x=w5832, y=w5839) -> (x*y=w5825:dbl)
                        n3151 = Multiply(x=w5831, y=w5838) -> (x*y=w5824:dbl)
                        n3152 = Multiply(x=w5830, y=w5837) -> (x*y=w5821:dbl)
                        n3153 = Multiply(x=w5829, y=w5836) -> (x*y=w5820:dbl)
                        n3154 = case shown="True" w5817 {
                          tunnel: w5825 -> [w5853 w5858]
                          tunnel: w5826 -> [_ w5856]
                          tunnel: [w5853 w5857] -> w5823
                          tunnel: w5824 -> [w5852 w5855]
                          tunnel: [w5852 w5854] -> w5822
                          frame False {
                          }
                          frame True {
                            n3155 = Multiply(x=w5856, y=w5855) -> (x*y=w5854:dbl)
                            n3156 = Multiply(x=w5856, y=w5858) -> (x*y=w5857:dbl)
                          }
                        }
                        n3157 = case shown="True" w5816 {
                          tunnel: w5821 -> [w5846 w5851]
                          tunnel: w5826 -> [_ w5849]
                          tunnel: [w5846 w5850] -> w5819
                          tunnel: w5820 -> [w5845 w5848]
                          tunnel: [w5845 w5847] -> w5818
                          frame False {
                          }
                          frame True {
                            n3158 = Multiply(x=w5849, y=w5848) -> (x*y=w5847:dbl)
                            n3159 = Multiply(x=w5849, y=w5851) -> (x*y=w5850:dbl)
                          }
                        }
                        n3160 = local read "SIG LAB02-2"() -> (w5841:T2)
                        n3161 = local read "SIG LAB02-1"() -> (w5843:T2)
                        n3162 = Bundle By Name(cluster=w5843, "Tmp Live"=w5823, "Tmp Neut"=w5822) -> (w5842:T2)
                        n3163 = Bundle By Name(cluster=w5841, "Tmp Live"=w5819, "Tmp Neut"=w5818) -> (w5840:T2)
                        n3164 = local write "SIG LAB02-1"(w5842) -> ()
                        n3165 = local write "SIG LAB02-2"(w5840) -> ()
                      }
                      frame 3 {
                        n3166 = case shown="False" w5873 {
                          tunnel: [w5904 w5905] -> w5889
                          tunnel: w5872 -> [_ w5905]
                          frame False {
                            n3167 = local read "CAL LAB03"() -> (w5904:T14)
                          }
                          frame True {
                          }
                        }
                        n3168 = local read "TEMP LA03"() -> (w5879:T9)
                        n3169 = local read "LAB03 TEMP"() -> (w5880:T12)
                        n3170 = call "sub vi - temperature delay v3.vi"("2-run"=w5861, "1-run"=w5862, "temp values IN"=w5879, "temp signals"=w5880) -> ("T2-N"=w5874:dbl, "T2-L"=w5875:dbl, "T1-N"=w5876:dbl, "T1-L"=w5877:dbl, "temp values OUT"=w5878:T44)  [unwired: 3 in]
                        n3171 = Unbundle By Name(w5889) -> ("1 (TL) cal"=w5884:dbl, "1 (TN) cal"=w5883:dbl, "2 (TL) cal"=w5882:dbl, "2 (TN) cal"=w5881:dbl)  [unwired: 6 out]
                        n3172 = local write "TEMP LA03"(w5878) -> ()
                        n3173 = Multiply(x=w5877, y=w5884) -> (x*y=w5870:dbl)
                        n3174 = Multiply(x=w5876, y=w5883) -> (x*y=w5869:dbl)
                        n3175 = Multiply(x=w5875, y=w5882) -> (x*y=w5866:dbl)
                        n3176 = Multiply(x=w5874, y=w5881) -> (x*y=w5865:dbl)
                        n3177 = case shown="True" w5861 {
                          tunnel: w5866 -> [w5891 w5896]
                          tunnel: w5871 -> [_ w5894]
                          tunnel: [w5891 w5895] -> w5864
                          tunnel: w5865 -> [w5890 w5893]
                          tunnel: [w5890 w5892] -> w5863
                          frame False {
                          }
                          frame True {
                            n3178 = Multiply(x=w5894, y=w5893) -> (x*y=w5892:dbl)
                            n3179 = Multiply(x=w5894, y=w5896) -> (x*y=w5895:dbl)
                          }
                        }
                        n3180 = case shown="True" w5862 {
                          tunnel: w5870 -> [w5898 w5903]
                          tunnel: w5871 -> [_ w5901]
                          tunnel: [w5898 w5902] -> w5868
                          tunnel: w5869 -> [w5897 w5900]
                          tunnel: [w5897 w5899] -> w5867
                          frame False {
                          }
                          frame True {
                            n3181 = Multiply(x=w5901, y=w5900) -> (x*y=w5899:dbl)
                            n3182 = Multiply(x=w5901, y=w5903) -> (x*y=w5902:dbl)
                          }
                        }
                        n3183 = local read "SIG LAB03-2"() -> (w5886:T2)
                        n3184 = local read "SIG LAB03-1"() -> (w5888:T2)
                        n3185 = Bundle By Name(cluster=w5888, "Tmp Live"=w5868, "Tmp Neut"=w5867) -> (w5887:T2)
                        n3186 = Bundle By Name(cluster=w5886, "Tmp Live"=w5864, "Tmp Neut"=w5863) -> (w5885:T2)
                        n3187 = local write "SIG LAB03-1"(w5887) -> ()
                        n3188 = local write "SIG LAB03-2"(w5885) -> ()
                      }
                      frame 4 {
                        n3189 = case shown="False" w5918 {
                          tunnel: [w5949 w5950] -> w5934
                          tunnel: w5917 -> [_ w5950]
                          frame False {
                            n3190 = local read "CAL LAB04"() -> (w5949:T14)
                          }
                          frame True {
                          }
                        }
                        n3191 = local read "LAB04 TEMP"() -> (w5924:T12)
                        n3192 = local read "TEMP LA04"() -> (w5925:T9)
                        n3193 = call "sub vi - temperature delay v3.vi"("2-run"=w5906, "1-run"=w5907, "temp values IN"=w5925, "temp signals"=w5924) -> ("T2-N"=w5919:dbl, "T2-L"=w5920:dbl, "T1-N"=w5921:dbl, "T1-L"=w5922:dbl, "temp values OUT"=w5923:T44)  [unwired: 3 in]
                        n3194 = Unbundle By Name(w5934) -> ("1 (TL) cal"=w5929:dbl, "1 (TN) cal"=w5928:dbl, "2 (TL) cal"=w5927:dbl, "2 (TN) cal"=w5926:dbl)  [unwired: 6 out]
                        n3195 = local write "TEMP LA04"(w5923) -> ()
                        n3196 = Multiply(x=w5922, y=w5929) -> (x*y=w5915:dbl)
                        n3197 = Multiply(x=w5921, y=w5928) -> (x*y=w5914:dbl)
                        n3198 = Multiply(x=w5920, y=w5927) -> (x*y=w5911:dbl)
                        n3199 = Multiply(x=w5919, y=w5926) -> (x*y=w5910:dbl)
                        n3200 = case shown="True" w5906 {
                          tunnel: w5911 -> [w5936 w5941]
                          tunnel: w5916 -> [_ w5939]
                          tunnel: [w5936 w5940] -> w5909
                          tunnel: w5910 -> [w5935 w5938]
                          tunnel: [w5935 w5937] -> w5908
                          frame False {
                          }
                          frame True {
                            n3201 = Multiply(x=w5939, y=w5938) -> (x*y=w5937:dbl)
                            n3202 = Multiply(x=w5939, y=w5941) -> (x*y=w5940:dbl)
                          }
                        }
                        n3203 = case shown="True" w5907 {
                          tunnel: w5915 -> [w5943 w5948]
                          tunnel: w5916 -> [_ w5946]
                          tunnel: [w5943 w5947] -> w5913
